vi "Initialize.vi"(8 "error in":errorcluster, 9 "INI File Path":path, 10 "Device":string) -> (0 "error out":errorcluster, 3 "Configuration out":refnum<class "Configuration.lvclass">)   [LabVIEW 2018, in "Configuration.lvlib" / "Configuration.lvclass"]
doc: "Load the configuration for the selected device from the config.ini file.\n\nWire INI Path for the exact project folder containing the config.ini file. Leave it empty for a C: drive search (legacy search 2020 or before)."
uses:
  Configuration.lvclass
  Configuration.lvclass/Configuration.ctl
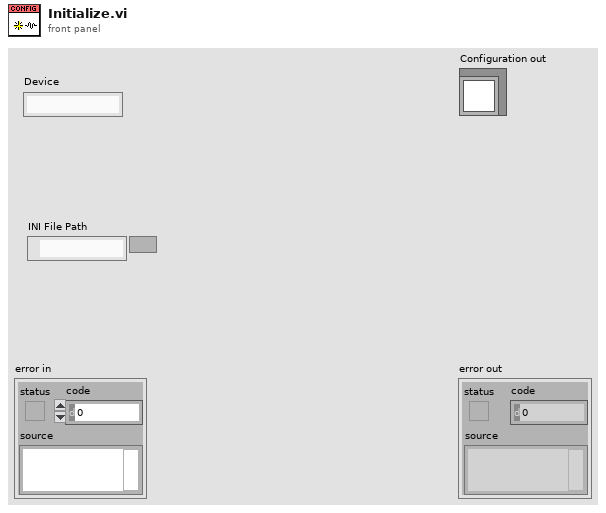
[diagram p1: front panel]
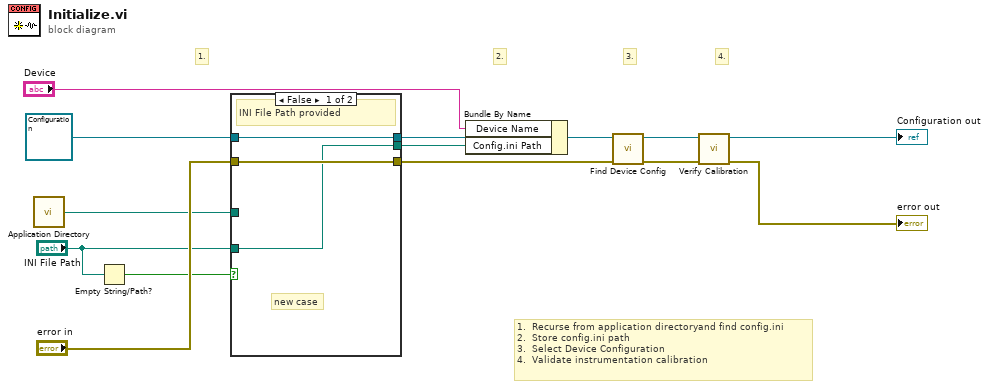
[diagram p0: block diagram]
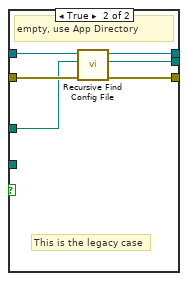
[diagram p2: hidden frame]
diagram:
  # "4."
  # "3."
  # "2."
  # "1."
  # "1.  Recurse from application directoryand find config.ini\n2.  Store config.ini path\n3.  Select Device Configuration\n4.  Validate instrumentation calibration"
  n1 = call <vilib>:"Application Directory.vi"() -> ("Application Directory"=w2:path)
  n2 = Empty String/Path?(string/path="INI File Path") -> (empty?=w3:bool)
  n3 = case shown="False" w3 {
    tunnel: refnum<class "Configuration.lvclass"> refnum ("Configuration in") -> [w17 w23]
    tunnel: [w17 w22] -> w12
    tunnel: [w15 w21] -> w11
    tunnel: "error in" -> [w16 w20]
    tunnel: [w16 w19] -> w9
    tunnel: w2 -> [_ w18]
    tunnel: "INI File Path" -> [w15 _]
    frame False {
      # "new case"
      # "INI File Path provided"
    }
    frame True {
      # "This is the legacy case"
      # "empty, use App Directory"
      n4 = call "Recursive Find Config File.vi"("error in"=w20, "Path"=w18, "Configuration in"=w23) -> ("error out"=w19:errorcluster, "File Path"=w21:path, "Configuration out"=w22:refnum<class "Configuration.lvclass">)  [unwired: 6 in]
    }
  }
  n5 = Bundle By Name(cluster=w12, "Device Name"="Device", "Config.ini Path"=w11) -> (w14:refnum<class "Configuration.lvclass">)
  n6 = call "Find Device Config.vi"("error in"=w9, "Configuration in"=w14) -> ("error out"=w5:errorcluster, "Configuration out"=w7:refnum<class "Configuration.lvclass">)  [unwired: 8 in]
  n7 = call "Verify Calibration.vi"("error in (no error)"=w5, "Configuration in"=w7) -> ("error out"=→"error out":errorcluster, "Configuration out"=→"Configuration out":refnum<class "Configuration.lvclass">)  [unwired: 8 in]
